vi "Cannon Get.vi"(1 "Stop Auto?":bool, 2 "Change Catcher":bool, 3 "Cannon Power":dbl) -> (0 "Cannon Info Out":T2)   [LabVIEW 2013]
uses:
  <vilib>/Rock Robotics/WPI/Solenoid/WPI_SolenoidValue.ctl
panel:
  # "Togle"
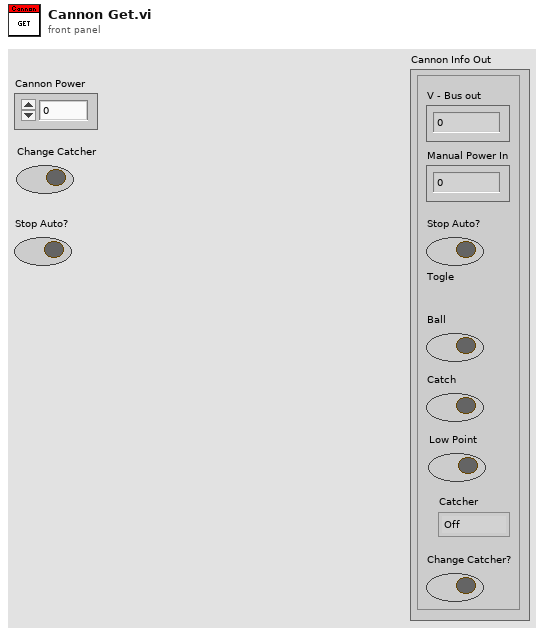
[diagram p1: front panel]
types:
  T1 = typedef "WPI_SolenoidValue.ctl" = enum16{"Off", "On", "Forward", "Reverse"}
  T2 = cluster{"V - Bus out":dbl, "Manual Power In":dbl, "Stop Auto?":bool, "Ball":bool, "Catch":bool, "Low Point":bool, "Catcher":T1, "Change Catcher?":bool}
  T3 = typedef "WPI_DigitalInputDevRef.ctl" = cluster{"DevStatus":errorcluster, "DIO Channel":T4, "Digital Module":T5}
  T4 = typedef "FPGA_DIOChannel.ctl" = enum8{"DIO 1", "DIO 2", "DIO 3", "DIO 4", "DIO 5", "DIO 6", "DIO 7", "DIO 8", "DIO 9", "DIO 10", "DIO 11", "DIO 12", "DIO 13", "DIO 14", "Invalid"}
  T5 = typedef "FPGA_TypedefDigitalModule.ctl" = enum16{"Digital Module 1", "Digital Module 2"}
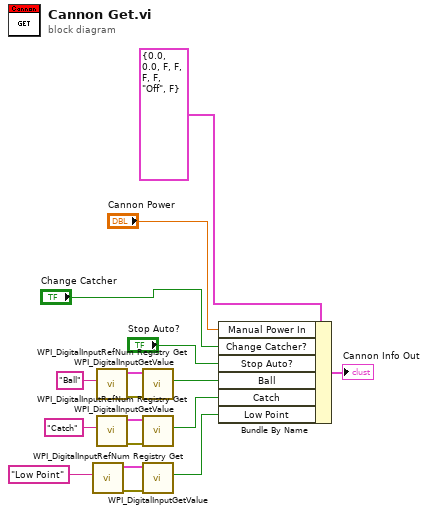
[diagram p0: block diagram]
diagram:
  n1 = call <vilib>:"WPI_DigitalInputRefNum Registry Get.vi"("refnum name"="Low Point") -> ("error out"=w8:errorcluster, "DigitalInputDevRef"=w7:T3)  [unwired: 9 in]
  n2 = call <vilib>:"WPI_DigitalInputRefNum Registry Get.vi"("refnum name"="Ball") -> ("error out"=w5:errorcluster, "DigitalInputDevRef"=w6:T3)  [unwired: 9 in]
  n3 = call <vilib>:"WPI_DigitalInputRefNum Registry Get.vi"("refnum name"="Catch") -> ("error out"=w10:errorcluster, "DigitalInputDevRef"=w9:T3)  [unwired: 9 in]
  n4 = call <vilib>:"WPI_DigitalInputGetValue.vi"("error in (no error)"=w5, "DigitalInputDevRef"=w6) -> ("Value"=w3:bool)  [unwired: 7 in, 2 out]
  n5 = call <vilib>:"WPI_DigitalInputGetValue.vi"("error in (no error)"=w10, "DigitalInputDevRef"=w9) -> ("Value"=w4:bool)  [unwired: 7 in, 2 out]
  n6 = call <vilib>:"WPI_DigitalInputGetValue.vi"("error in (no error)"=w8, "DigitalInputDevRef"=w7) -> ("Value"=w2:bool)  [unwired: 7 in, 2 out]
  n7 = Bundle By Name(cluster=T2 {"V - Bus out"=0.0, "Manual Power In"=0.0, "Stop Auto?"=FALSE, "Ball"=FALSE, "Catch"=FALSE, "Low Point"=FALSE, "Catcher"=enum."Off", "Change Catcher?"=FALSE} ("Cannon Info Out"), "Manual Power In"="Cannon Power", "Change Catcher?"="Change Catcher", "Stop Auto?"="Stop Auto?", "Ball"=w3, "Catch"=w4, "Low Point"=w2) -> (→"Cannon Info Out":T2)
